vi "_FPGA_Avg1024Elememts_I16.vi"(3 "Start_latch":bool, 4 "Enable":bool, 5 "I16 in":i16) -> (0 "Updating":bool, 2 "Avg I16":i16)   [LabVIEW 2018]
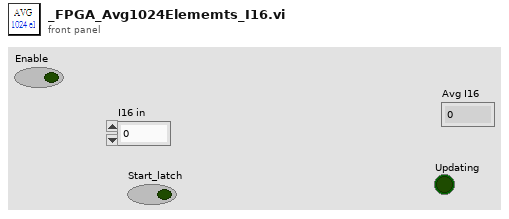
[diagram p1: front panel]
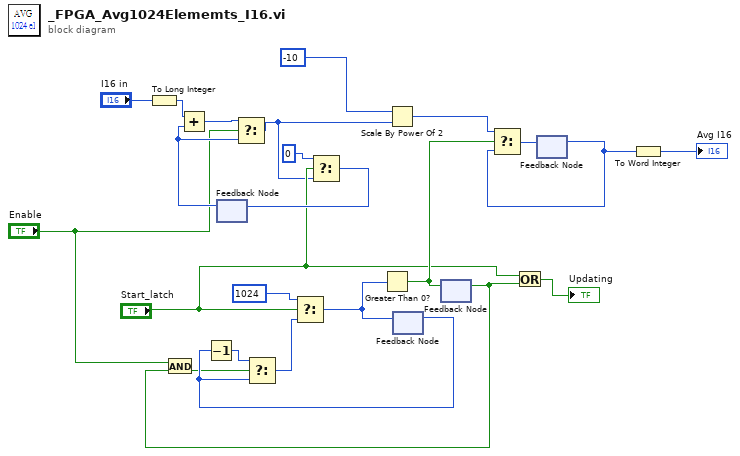
[diagram p0: block diagram]
diagram:
  n1 = To Long Integer(number="I16 in") -> (32bit integer=w22:i32)
  n2 = feedback #1() -> (w3:i32)  [unwired: 1 in]
  n3 = Add(x=w22, y=w3) -> (x+y=w4:i32)
  n4 = Select(t=w4, s="Enable", f=w3) -> (s? t:f=w5:i32)
  n5 = Select(t=0, s="Start_latch", f=w5) -> (s? t:f=w8:i32)
  n6 = feedback-in #1(w8) -> ()
  n7 = Scale By Power Of 2(n=i16 -10, x=w5) -> (x*2^n=w15:i32)
  n8 = feedback #2() -> (w17:u16)  [unwired: 1 in]
  n9 = Decrement(x=w17) -> (x-1=w18:u16)
  n10 = feedback #3() -> (w12:bool)  [unwired: 1 in]
  n11 = And(x="Enable", y=w12) -> (x .and. y?=w2:bool)
  n12 = Select(t=w18, s=w2, f=w17) -> (s? t:f=w16:u16)
  n13 = Select(t=u16 1024, s="Start_latch", f=w16) -> (s? t:f=w19:u16)
  n14 = Greater Than 0?(x=w19) -> (x > 0?=w11:bool)
  n15 = feedback-in #2(w19) -> ()
  n16 = feedback-in #3(w11) -> ()
  n17 = Or(x="Start_latch", y=w12) -> (x .or. y?=→"Updating":bool)
  n18 = feedback #4() -> (w10:i32)  [unwired: 1 in]
  n19 = Select(t=w15, s=w11, f=w10) -> (s? t:f=w14:i32)
  n20 = feedback-in #4(w14) -> ()
  n21 = To Word Integer(number=w10) -> (16bit integer=→"Avg I16":i16)
